vi "Dispose Module Images.vi"(8 "error in":errorcluster, 11 "Potting Procedure in":refnum<class "Potting Procedure.lvclass">) -> (0 "error out":errorcluster, 3 "Potting Procedure out":refnum<class "Potting Procedure.lvclass">)   [LabVIEW 2011, in "Potting Procedure.lvclass"]
uses:
  Potting Procedure.lvclass
  <vilib>/vision/Image Controls.llb/IMAQ Image.ctl
  Shared Components/Vec3d Class/Vec3d Class.lvclass
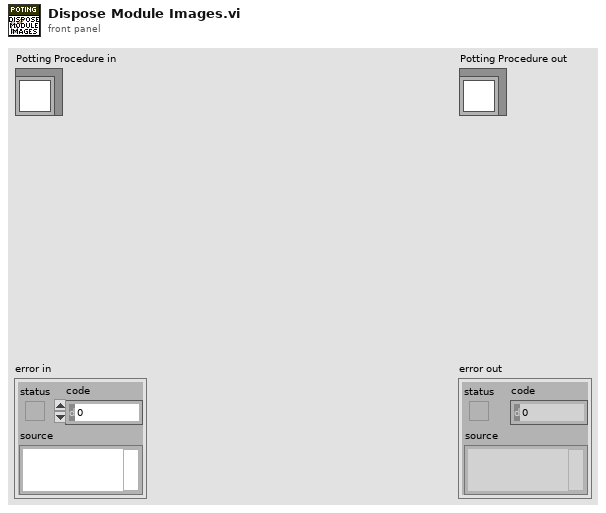
[diagram p1: front panel]
types:
  T1 = typedef "IMAQ Image.ctl" = refnum<image>
  T2 = typedef "Inspect Modules.ctl" = cluster{"Has Been Run?":bool, "Module Positions":cluster{"TBM-TBM":T3, "TBM-HDI":T3, "Address Pads":T3, "HDI Bond Pad References":T6[], "BBM Bond Pad References":T6[], "HV-HDI":T6, "HV-BBM":T6, "Chuck":i32, "Slot":i32}[]}
  T3 = typedef "Multi-Fiducial Image.ctl" = cluster{"Fiducial Image":T4, "Fiducials":cluster{"Selected Fiducial":T5, "fiducial name":string}[]}
  T4 = typedef "Physical Image.ctl" = cluster{"Image Position":refnum<class "Vec3d Class.lvclass">, "Image Reference":T1, "Field of View":cluster{"x(mm)":dbl, "y(mm)":dbl}}
  T5 = typedef "Fiducial with Source.ctl" = cluster{"Fiducial Image Coordinate":refnum<class "Vec3d Class.lvclass">, "Fiducial Source":enum16{"Pattern Recognition", "User", "Error", "Default"}}
  T6 = typedef "Fiducial Image.ctl" = cluster{"Fiducial Image":T4, "Selected Fiducial":T5, "fiducial name":string}
  T7 = cluster{"TBM-TBM":T3, "TBM-HDI":T3, "Address Pads":T3, "HDI Bond Pad References":T6[], "BBM Bond Pad References":T6[], "HV-HDI":T6, "HV-BBM":T6, "Chuck":i32, "Slot":i32}[]
  T8 = cluster{"TBM-TBM":T3, "TBM-HDI":T3, "Address Pads":T3, "HDI Bond Pad References":T6[], "BBM Bond Pad References":T6[], "HV-HDI":T6, "HV-BBM":T6, "Chuck":i32, "Slot":i32}
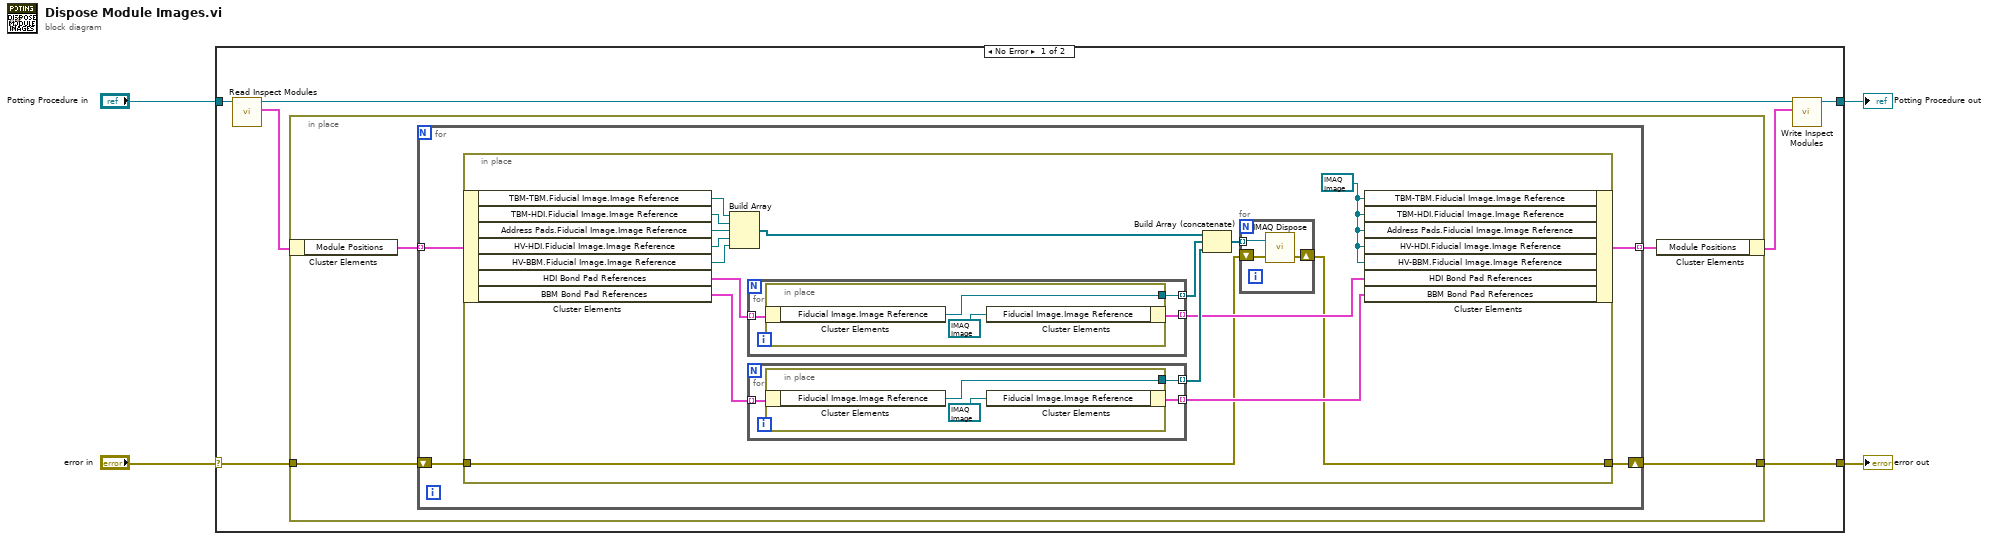
[diagram p0: block diagram]
diagram:
  n1 = case shown="No Error" "error in" {
    selector: "error in" -> [w6 w50]
    tunnel: [w5 w50] -> w3
    tunnel: [w7 w49] -> w1
    tunnel: "Potting Procedure in" -> [w11 w49]
    frame No Error {
      n2 = call-dynamic "Read Inspect Modules.vi"("Potting Procedure in"=w11) -> ("Inspect Modules"=w10:T2, "Potting Procedure out"=w8:refnum<class "Potting Procedure.lvclass">)  [unwired: 8 in, 1 out]
      n3 = in-place {
        in-place-border: w6 -> [w13]
        in-place-border: [w12] -> w5
        n4 = in-place-cluster #1(w10) -> ("Module Positions"=w15:T7)
        n5 = for {
          tunnel: w15 -> [w19] mode=indexing
          tunnel: [w18] -> w14 mode=indexing
          shift-right: [w16] -> w12
          shift-left: w13 -> [w17]
          n6 = in-place {
            in-place-border: w17 -> [w21]
            in-place-border: [w20] -> w16
            w35 = T1 refnum ("TBM-TBM.Fiducial Image.Image Reference")
            n7 = in-place-cluster #2(w19) -> ("TBM-TBM.Fiducial Image.Image Reference"=w34:T1, "TBM-HDI.Fiducial Image.Image Reference"=w33:T1, "Address Pads.Fiducial Image.Image Reference"=w32:T1, "HV-HDI.Fiducial Image.Image Reference"=w31:T1, "HV-BBM.Fiducial Image.Image Reference"=w30:T1, "HDI Bond Pad References"=w27:T6[], "BBM Bond Pad References"=w26:T6[])
            n8 = Build Array(w34, w33, w32, w31, w30) -> (w29:T1[])
            n9 = for {
              tunnel: w27 -> [w46] mode=indexing
              tunnel: [w45] -> w28 mode=indexing
              tunnel: [w44] -> w24 mode=indexing
              n10 = in-place {
                in-place-border: [w47] -> w45
                n11 = in-place-cluster #3(w46) -> ("Fiducial Image.Image Reference"=w47:T1)
                n12 = in-place-cluster #3("Fiducial Image.Image Reference"=T1 refnum) -> (w44:T6)
              }
            }
            n13 = for {
              tunnel: w26 -> [w41] mode=indexing
              tunnel: [w40] -> w25 mode=indexing
              tunnel: [w39] -> w23 mode=indexing
              n14 = in-place {
                in-place-border: [w42] -> w40
                n15 = in-place-cluster #4(w41) -> ("Fiducial Image.Image Reference"=w42:T1)
                n16 = in-place-cluster #4("Fiducial Image.Image Reference"=T1 refnum) -> (w39:T6)
              }
            }
            n17 = Build Array (concatenate)(w29, w28, w25) -> (w22:T1[])
            n18 = for {
              tunnel: w22 -> [w38] mode=indexing
              shift-right: [w36] -> w20
              shift-left: w21 -> [w37]
              n19 = call "IMAQ Dispose"("Image"=w38, "error in (no error)"=w37) -> ("error out"=w36:errorcluster)  [unwired: 4 in]
            }
            n20 = in-place-cluster #2("TBM-TBM.Fiducial Image.Image Reference"=w35, "TBM-HDI.Fiducial Image.Image Reference"=w35, "Address Pads.Fiducial Image.Image Reference"=w35, "HV-HDI.Fiducial Image.Image Reference"=w35, "HV-BBM.Fiducial Image.Image Reference"=w35, "HDI Bond Pad References"=w24, "BBM Bond Pad References"=w23) -> (w18:T8)
          }
        }
        n21 = in-place-cluster #1("Module Positions"=w14) -> (w9:T2)
      }
      n22 = call-dynamic "Write Inspect Modules.vi"("Inspect Modules"=w9, "Potting Procedure in"=w8) -> ("Potting Procedure out"=w7:refnum<class "Potting Procedure.lvclass">)  [unwired: 8 in, 1 out]
    }
    frame Error {
    }
  }
  "error out" <- w3
  "Potting Procedure out" <- w1
